vi "GlobalReservedNames.vi"() -> ()   [LabVIEW 2013]
panel:
  in  "ReservedNames":string[](array[string])=["t", "f", "tMax", "dt", "and", "break", "do", "else", "elseif", "end", "false", "for", "function", "if", "in", "local", "nil", "not", "or", "repeat", "return", "then", "true", "until", "while"]
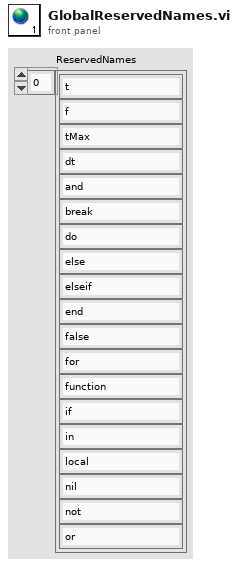
[diagram p1: front panel]
diagram:
